vi "6009 Voice Acquisition.vi"() -> ()   [LabVIEW 2015]
uses:
  <vilib>/Analysis/4window.llb/windowTd.ctl
  <vilib>/measure/maspectr.llb/Power Spectrum and PSD Export Mode.ctl
  <vilib>/DAQmx/read.llb/DAQmx Read (Analog Wfm 1Chan NSamp).vi
  <vilib>/DAQmx/miscellaneous.llb/DAQmx Fill In Error Info.vi
  <vilib>/measure/maspectr.llb/FFT Power Spectrum and PSD for 1 Chan.vi
  <vilib>/measure/maspectr.llb/FFT Spectrum (Mag-Phase) for 1 Chan.vi
  <vilib>/measure/matone.llb/Harmonic Distortion Analyzer 1 Chan.vi
  <vilib>/measure/NI_MAPro.lvlib
  <vilib>/Analysis/NI_AALPro.lvlib
panel:
  out "Power Spectrum / PSD":cluster{"f0":dbl, "df":dbl, "magnitude":dbl[]} {"magnitude" format="%.2p"; "f0" format="%0.2p"; "df" format="%0.2p"}
  in  "Export to Excel":bool
  in  "Execution Selector":bool
  in  "Tab Control":T1(tab)
  out "Power FFT":cluster{"f0":dbl, "df":dbl, "magnitude":dbl[]}(graph)
  out "f0":dbl
  out "df":dbl
  out "Max Freq (Hz)":dbl
  out "Raw magnitude":dbl[](array[numeric])
  out "Filtered output array":dbl[](array[numeric])
  out "Max Freq (Hz)":dbl
  out "Filtered output":dbl[](array[numeric])
  out "PSD FFT":cluster{"f0":dbl, "df":dbl, "magnitude":dbl[]}(graph)
  out "PSD magnitude":dbl[](array[numeric])
  out "df":dbl
  out "f0":dbl
  out "Power FFT (controllable)":cluster{"f0":dbl, "df":dbl, "magnitude":dbl[]}(graph)
  in  "FFT METHOD":T2=62 items=["Rectangle"=0, "Hanning"=1, "Hamming"=2, "Blackman-Harris"=3, "Exact Blackman"=4, "Blackman"=5, "Flat Top"=6, "4 Term B-Harris "=7, "7 Term B-Harris"=8, "Low Sidelobe"=9, "Blackman Nuttall"=11, "Triangle"=30, "Bartlett-Hanning"=31, "Bohman"=32, "Parzen"=33, "Welch"=34, "Kaiser"=60, "Dolph-Chebyshev"=61, "Gaussian"=62]
  out "Spectrum Data":T3(graph)
  out "fundamental frequency":dbl format="%.2p"
  in  "export mode":T4(ring)=enum."fundamental signal"
  in  "stop":bool
  out "error out":errorcluster
  in  "error in":errorcluster
  # "ENGR 301 - Analog Audio Spectrum Analysis"
  # "Use the control below to select from various algorithms\nused to create FFT waveform graphs."
  # "Use the control below to select from various display\noptions for this analysis method."
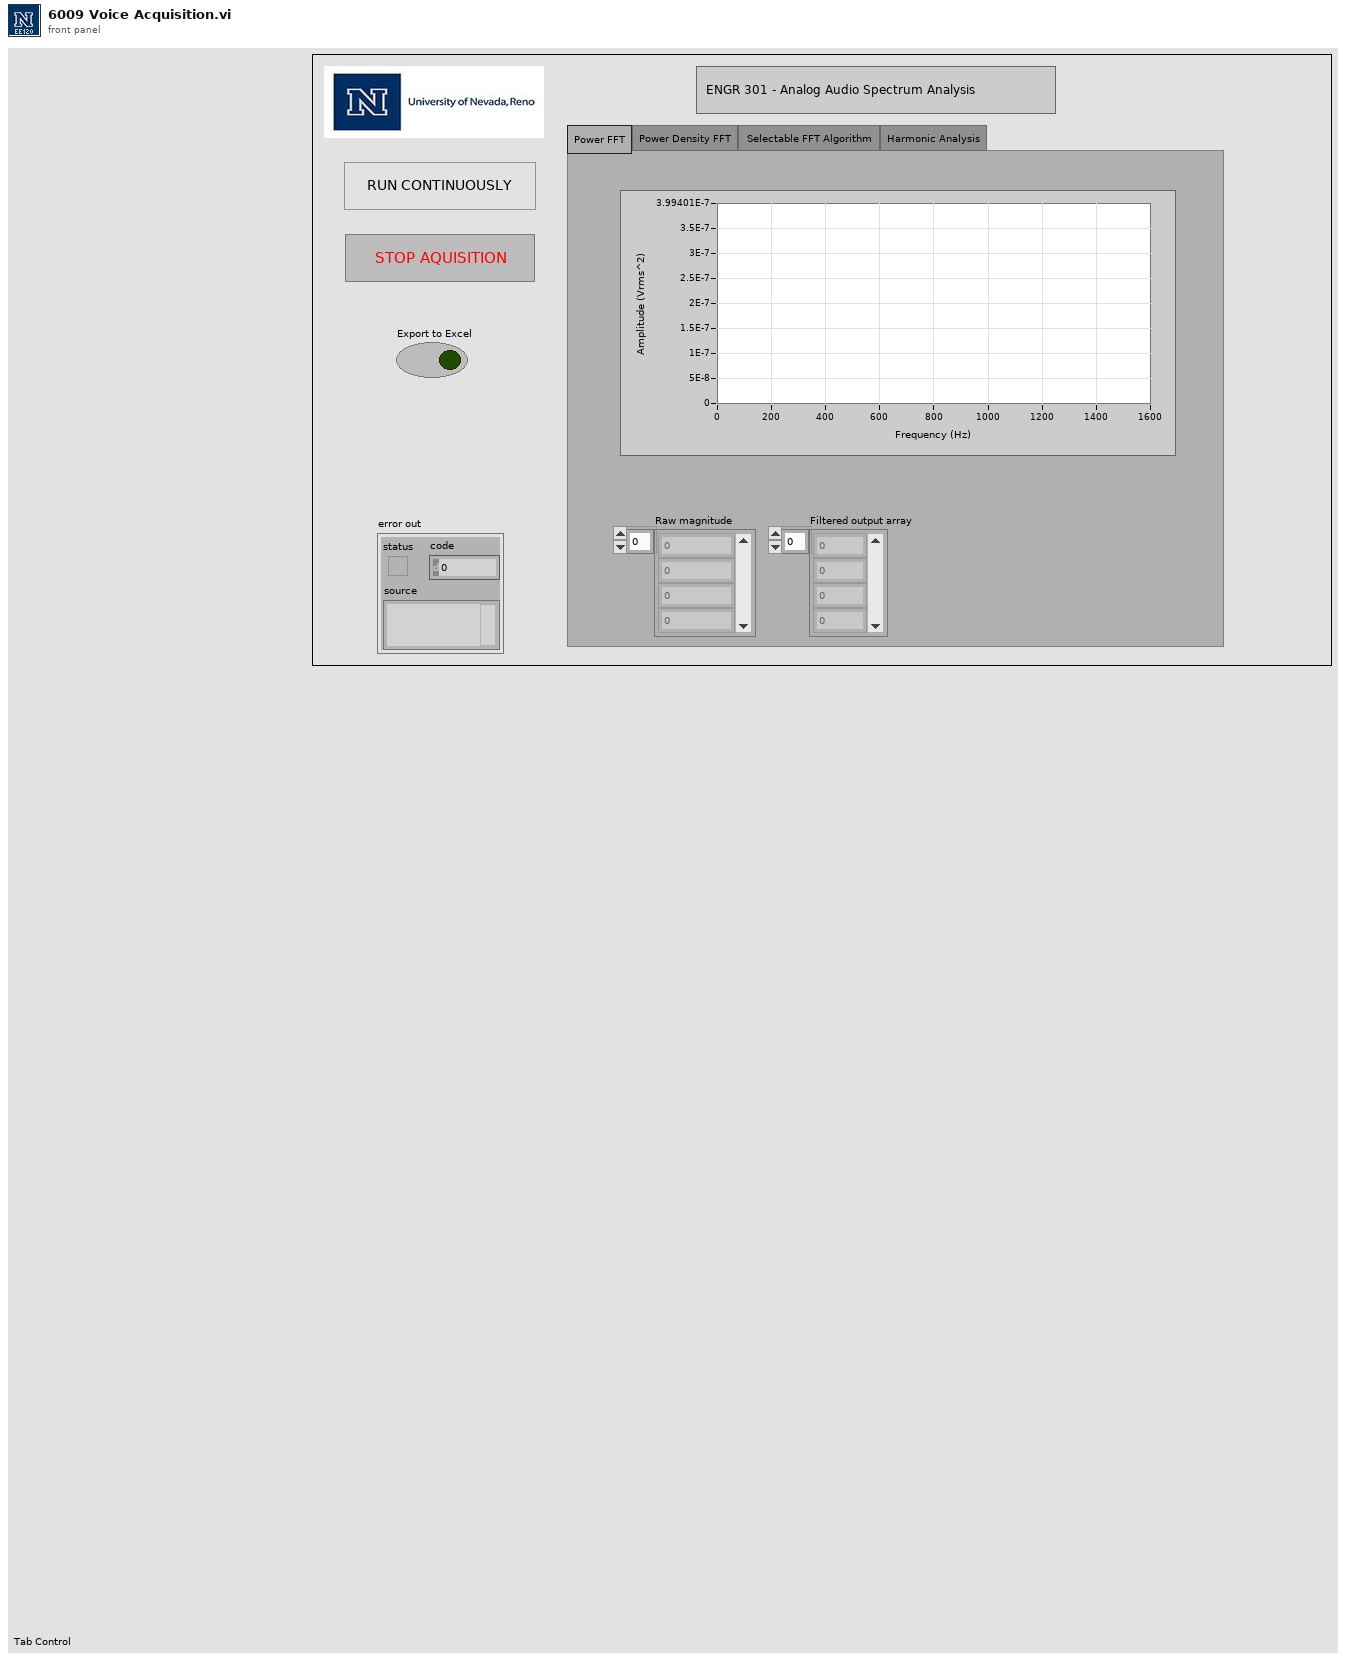
[diagram p1: front panel]
types:
  T1 = enum32{"Power FFT", "Power Density FFT", "Selectable FFT Algorithm ", "Harmonic Analysis"}
  T2 = typedef "NI_AALPro.lvlib/windowTd.ctl" = u32
  T3 = cluster{"f0":dbl, "df":dbl, "dB Spectrum (Hann)":dbl[]}
  T4 = enum16{"none", "input signal", "fundamental signal", "residual signal", "harmonics only", "noise and spurs"}
  T5 = typedef "NI_MAPro.lvlib/Power Spectrum and PSD Export Mode.ctl" = u16
  T6 = cluster{"exported time signal":waveform(dbl), "exported spectrum (dB)":cluster{"f0":dbl, "df":dbl, "dB Spectrum (Hann)":dbl[]}}
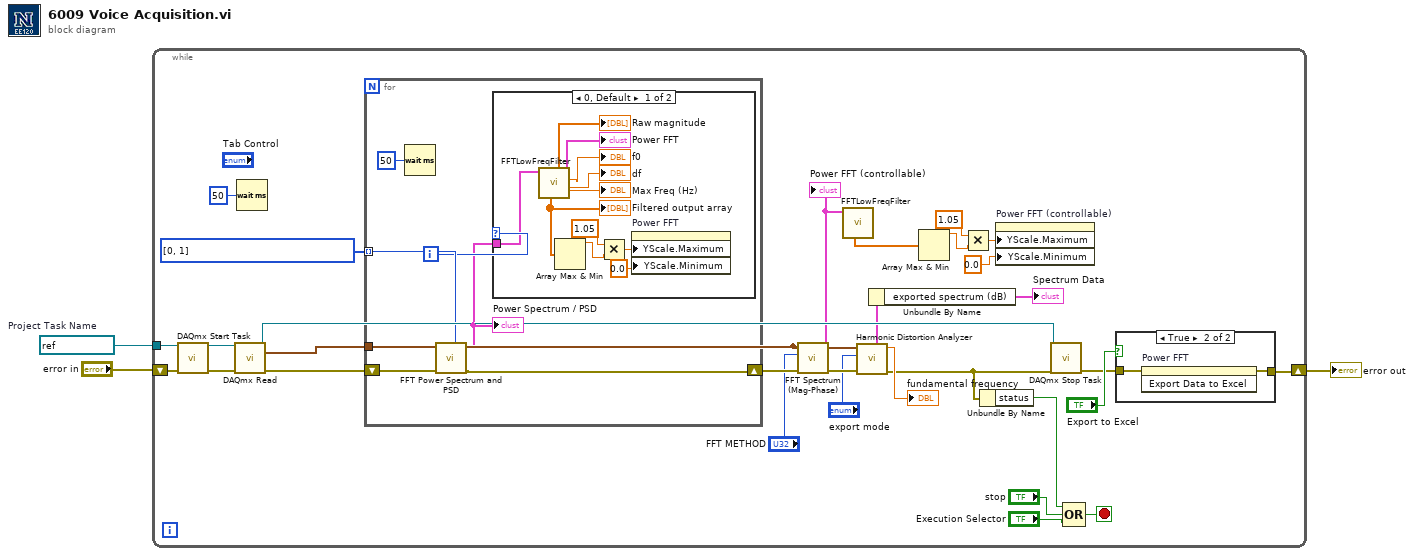
[diagram p0: block diagram]
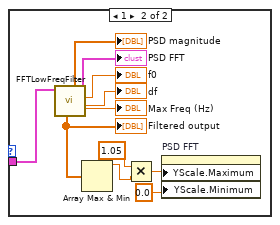
[diagram p3: hidden frame]
diagram:
  w3 = refnum<k21> "Audio IN"  # Project Task Name
  n1 = while {
    shift-right: [w5] -> w1
    shift-left: "error in" -> [w11]
    tunnel: w3 -> [w10]
    stop <- w20 stop-if-true
    w19 = T5[] [0, 1] items=["Power Spectrum", "Power Spectral Density"] ("FFT Method")
    n2 = call <vilib>:"DAQmx Start Task.vi"("task/channels in"=w10, "error in"=w11) -> ("task out"=w12:refnum<k21>, "error out"=w13:errorcluster)  [unwired: 12 in]
    n3 = call-poly <vilib>:"DAQmx Read.vi"("task/channels in"=w12, "error in"=w13) -> ("task out"=w30:refnum<k21>, "data"=w4:waveform(dbl), "error out"=w8:errorcluster)  [unwired: 11 in]
    n4 = Wait (ms)(milliseconds to wait=u32 50) -> ()  [unwired: 1 out]
    n5 = for {
      shift-right: [w37] -> w33
      shift-left: w8 -> [w43]
      tunnel: w19 -> [w42] mode=indexing
      tunnel: w4 -> [w39]
      i -> [w41]
      n6 = Wait (ms)(milliseconds to wait=u32 50) -> ()  [unwired: 1 out]
      n7 = call-poly <vilib>:"FFT Power Spectrum and PSD.vi"("export mode"=w42, "error in (no error)"=w43, "time signal"=w39) -> ("error out"=w37:errorcluster, "Power Spectrum / PSD"=w38:cluster{"f0":dbl, "df":dbl, "magnitude":dbl[]})  [unwired: 5 in, 2 out]
      "Power Spectrum / PSD" <- w38
      n8 = case shown="0, Default" w41 {
        tunnel: w38 -> [w50 w60]
        frame 0, Default {
          n9 = call "FFTLowFreqFilter.vi"("Power Spectrum / PSD"=w50) -> ("df"=→"df":dbl, "f0"=→"f0":dbl, "Power FFT"=→"Power FFT":cluster{"f0":dbl, "df":dbl, "magnitude":dbl[]}, "Max Freq (Hz)"=→"Max Freq (Hz)":dbl, "Raw magnitude"=→"Raw magnitude":dbl[], "Filtered output array"=w46:dbl[])  [unwired: 5 in]
          "Filtered output array" <- w46
          n10 = Array Max & Min(array=w46) -> (max value=w48:dbl)  [unwired: 3 out]
          n11 = Multiply(x=1.05, y=w48) -> (x*y=w49:dbl)
          n12 = property on="Power FFT" class="WFGraph (strict)"("YScale.Maximum"=w49, "YScale.Minimum"=0.0 ("Y Scale.Range:Minimum")) -> ()  [unwired: 2 in, 2 out]
        }
        frame 1 {
          n13 = call "FFTLowFreqFilter.vi"("Power Spectrum / PSD"=w60) -> ("df"=→"df":dbl, "f0"=→"f0":dbl, "Power FFT"=→"PSD FFT":cluster{"f0":dbl, "df":dbl, "magnitude":dbl[]}, "Max Freq (Hz)"=→"Max Freq (Hz)":dbl, "Raw magnitude"=→"PSD magnitude":dbl[], "Filtered output array"=w59:dbl[])  [unwired: 5 in]
          "Filtered output" <- w59
          n14 = Array Max & Min(array=w59) -> (max value=w58:dbl)  [unwired: 3 out]
          n15 = Multiply(x=1.05, y=w58) -> (x*y=w56:dbl)
          n16 = property on="PSD FFT" class="WFGraph (strict)"("YScale.Maximum"=w56, "YScale.Minimum"=0.0 ("Y Scale.Range:Minimum")) -> ()  [unwired: 2 in, 2 out]
        }
      }
    }
    n17 = call-poly <vilib>:"FFT Spectrum (Mag-Phase).vi"("error in (no error)"=w33, "window"="FFT METHOD", "time signal"=w4) -> ("error out"=w29:errorcluster, "magnitude"=w15:cluster{"f0":dbl, "df":dbl, "magnitude":dbl[]})  [unwired: 4 in, 3 out]
    "Power FFT (controllable)" <- w15
    n18 = call "FFTLowFreqFilter.vi"("Power Spectrum / PSD"=w15) -> ("Filtered output array"=w14:dbl[])  [unwired: 5 in, 5 out]
    n19 = call-poly <vilib>:"Harmonic Distortion Analyzer.vi"("error in (no error)"=w29, "export mode"="export mode", "signal in"=w4) -> ("error out"=w24:errorcluster, "detected fundamental frequency"=→"fundamental frequency":dbl, "exported signals"=w28:T6)  [unwired: 3 in, 3 out]
    n20 = Unbundle By Name(w28) -> ("exported spectrum (dB)"=→"Spectrum Data":T3)
    n21 = Array Max & Min(array=w14) -> (max value=w17:dbl)  [unwired: 3 out]
    n22 = Multiply(x=1.05, y=w17) -> (x*y=w16:dbl)
    n23 = Unbundle By Name(w24) -> ("status"=w23:bool)
    n24 = property on="Power FFT (controllable)" class="WFGraph (strict)"("YScale.Maximum"=w16, "YScale.Minimum"=0.0 ("Y Scale.Range:Minimum")) -> ()  [unwired: 2 in, 2 out]
    n25 = call <vilib>:"DAQmx Stop Task.vi"("task/channels in"=w30, "error in"=w24) -> ("error out"=w6:errorcluster)  [unwired: 12 in, 1 out]
    n26 = Compound Arithmetic op=OR(w23, "stop", "Execution Selector") -> (w20:bool)
    n27 = case shown="True" "Export to Excel" {
      tunnel: [w34 w35] -> w5
      tunnel: w6 -> [w34 w36]
      frame False {
      }
      frame True {
        n28 = invoke on="Power FFT" class="WFGraph (strict)" method="Export Data to Excel"(error in=w36) -> (error out=w35:errorcluster)  [unwired: 2 in, 2 out]
      }
    }
  }
  "error out" <- w1
